vi "DAC Configure.vi"(8 "error in":errorcluster, 11 "DAC TEG Temp in":refnum<class "DAC TEG Temp.lvclass">) -> (0 "error out":errorcluster, 3 "DAC TEG Temp out":refnum<class "DAC TEG Temp.lvclass">)   [LabVIEW 2019, in "DAC.lvlib" / "DAC TEG Temp.lvclass"]
uses:
  DAC TEG Temp.lvclass
  C:/Users/krio/Documents/LV_Projects/test-stand/App/DAC/DAC.lvclass
  DAC.lvclass/DAC.ctl
  DAC TEG Temp.lvclass/DAC TEG Temp.ctl
  <vilib>/Instr/_visa.llb/VISA Configure Serial Port (Instr).vi
  DAC.lvclass
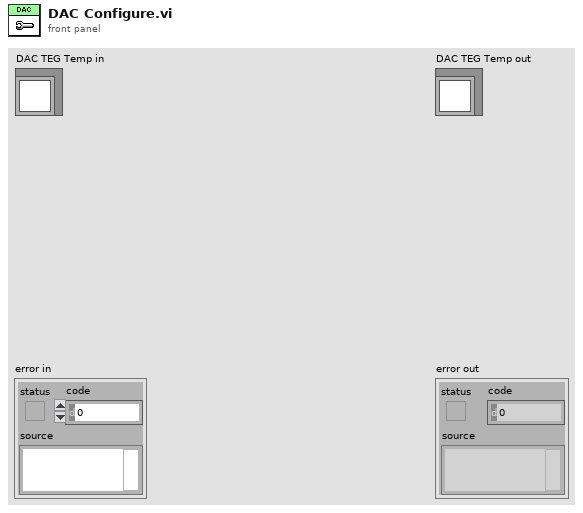
[diagram p1: front panel]
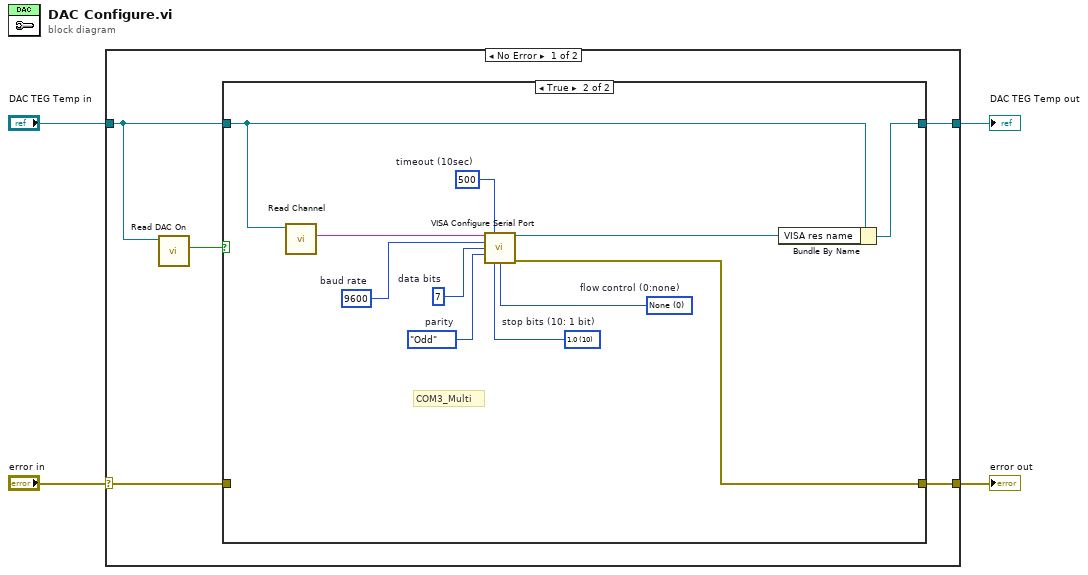
[diagram p0: block diagram]
diagram:
  n1 = case shown="No Error" "error in" {
    selector: "error in" -> [w6 w24]
    tunnel: [w5 w24] -> w4
    tunnel: [w7 w23] -> w3
    tunnel: "DAC TEG Temp in" -> [w9 w23]
    frame No Error {
      n2 = call "Read DAC On.vi"("DAC in"=w9) -> ("DAC On"=w8:bool)  [unwired: 8 in, 2 out]
      n3 = case shown="True" w8 {
        tunnel: w9 -> [w11 w21]
        tunnel: [w11 w22] -> w7
        tunnel: w6 -> [w10 _]
        tunnel: [w10 w12] -> w5
        frame False {
        }
        frame True {
          w15 = u16 0 items=["None", "XON/XOFF", "RTS/CTS", "XON/XOFF & RTS/CTS", "DTR/DSR", "XON/XOFF & DTR/DSR"]  # flow control (0:none)
          w16 = u16 10 items=["1.0"=10, "1.5"=15, "2.0"=20]  # stop bits (10: 1 bit)
          w17 = enum16{"None", "Odd", "Even", "Mark", "Space"}."Odd"  # parity
          w18 = u16 7  # data bits
          w19 = u32 9600  # baud rate
          w20 = u32 500  # timeout (10sec)
          # "COM3_Multi"
          n4 = call "Read Channel.vi"("DAC in"=w21) -> ("Channel"=w14:string)  [unwired: 8 in, 2 out]
          n5 = call-poly "VISA Configure Serial Port"("VISA resource name"=w14, "timeout (10sec)"=w20, "baud rate (9600)"=w19, "data bits (8)"=w18, "parity (0:none)"=w17, "stop bits (10: 1 bit)"=w16, "flow control (0:none)"=w15) -> ("VISA resource name out"=w13:refnum<visa-resource-name>, "error out"=w12:errorcluster)  [unwired: 7 in]
          n6 = Bundle By Name(cluster=w21, "VISA res name"=w13) -> (w22:refnum<class "DAC TEG Temp.lvclass">)
        }
      }
    }
    frame Error {
    }
  }
  "error out" <- w4
  "DAC TEG Temp out" <- w3
